vi "MD5 (File).vi"(10 "filepath":path) -> (2 "MD5 hash":string)   [LabVIEW 2024, in "MD5.lvlib"]
uses:
  MD5.lvlib
  Data-vector.ctl
  MD5.lvclass
  pad.vi
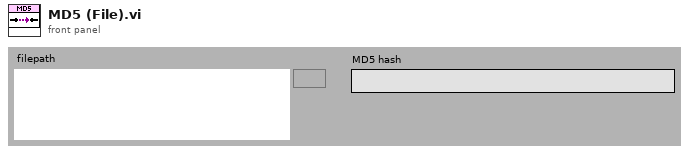
[diagram p1: front panel]
types:
  T1 = typedef "MD5.lvlib/MD5.lvclass/Data-vector.ctl" = cluster{"Data[ ]":u8[], "end":bool}
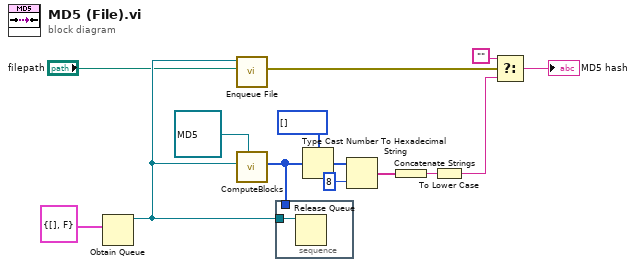
[diagram p0: block diagram]
diagram:
  n1 = Obtain Queue(element data type=T1 {"Data[ ]"=[], "end"=FALSE} ("cluster")) -> (queue out=w11:refnum<queue>)  [unwired: 4 in, 2 out]
  n2 = call "Enqueue File.vi"("filepath"="filepath", "Blocks queue"=w11) -> ("error out"=w9:errorcluster)  [unwired: 9 in]
  n3 = call-dynamic "ComputeBlocks.vi"("MD5"=refnum<class "MD5.lvclass"> refnum ("SHA-1"), "blocks queue"=w11) -> ("hash"=w7:u8[])  [unwired: 9 in]
  n4 = stacked-sequence {
    tunnel: w11 -> [w15]
    tunnel: w7 -> [_]
    frame #0 {
      n5 = Release Queue(queue=w15) -> ()  [unwired: 2 in, 3 out]
    }
  }
  n6 = Type Cast(type=u32[] [] ("U32"), x=w7) -> (*(type *) &x=w5:u32[])
  n7 = Number To Hexadecimal String(1:i16 8 ("width (-)"), 2:w5) -> (0:w4:string[])
  n8 = Concatenate Strings(w4) -> (w3:string)
  n9 = To Lower Case(string=w3) -> (all lower case string=w1:string)
  n10 = Select(t="", s=w9, f=w1) -> (s? t:f=→"MD5 hash":string)
